vi "SeqWithMultichannel.vi"() -> ()   [LabVIEW 2014]
uses:
  <vilib>/Instr/_visa.llb/VISA Configure Serial Port (Instr).vi
panel:
  out "read buffer":string
  out "OutputStr":string
  in  "stop":bool
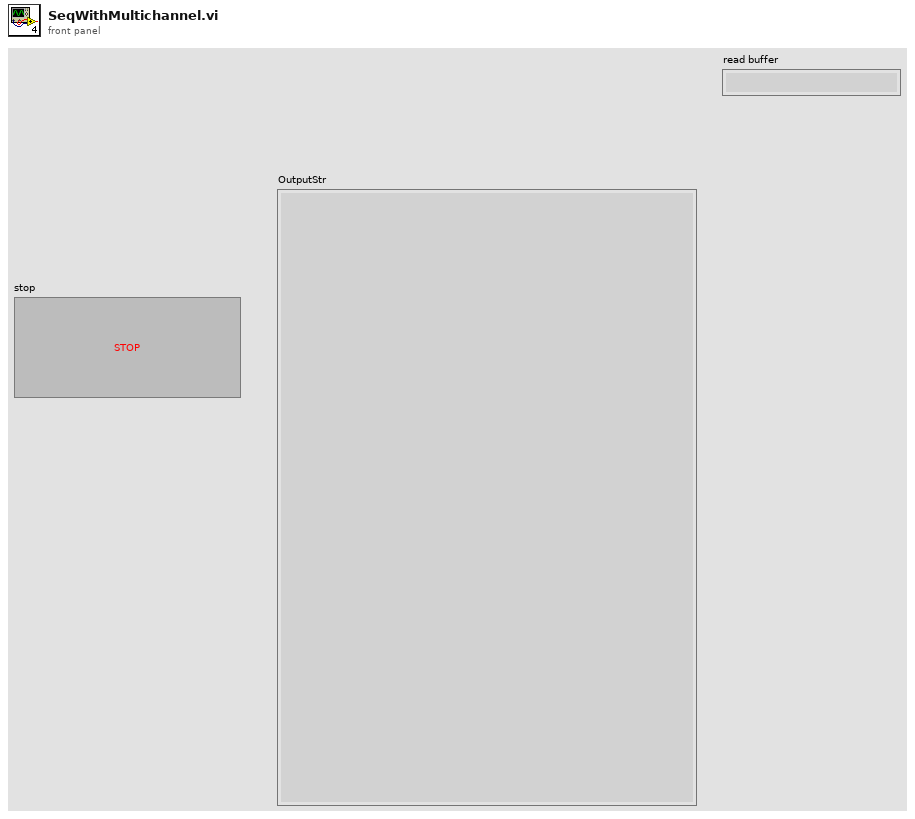
[diagram p1: front panel]
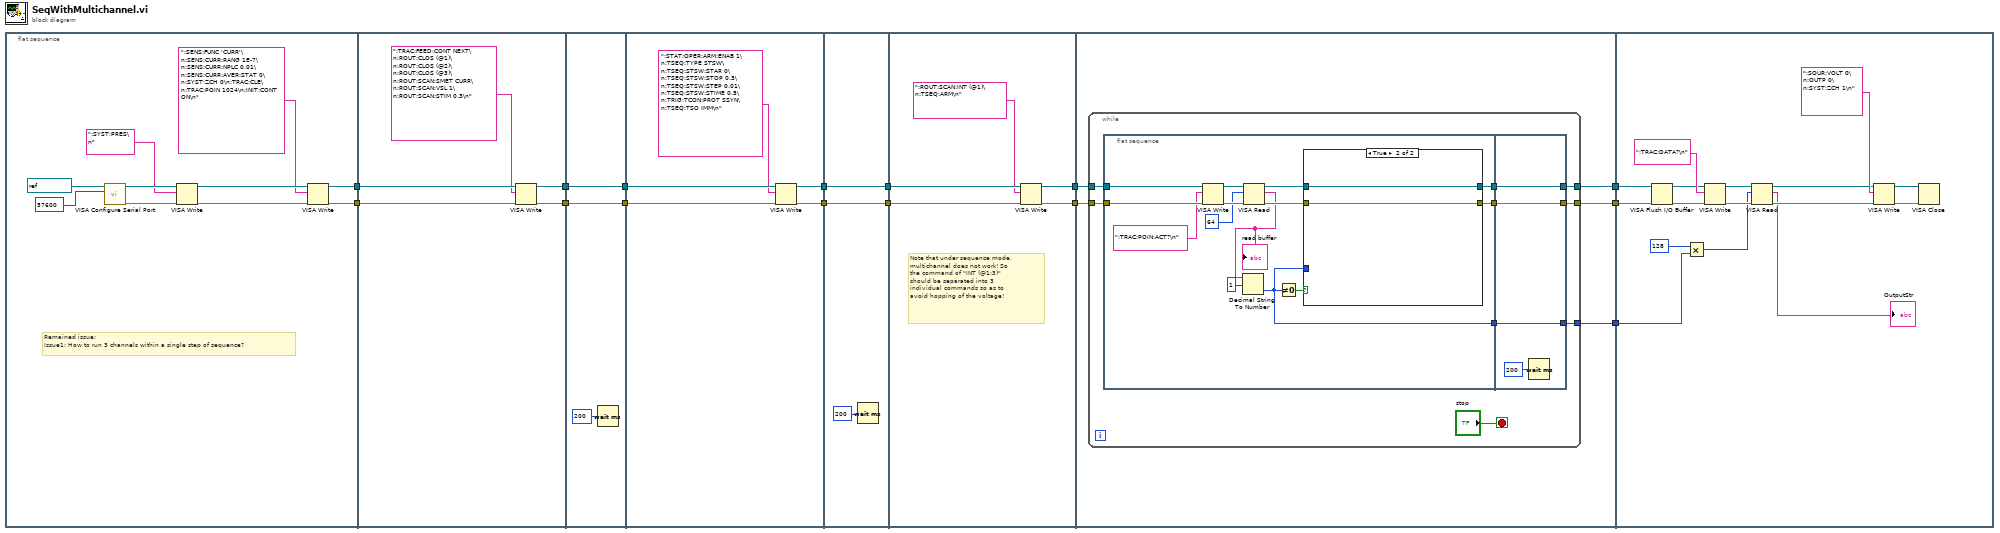
[diagram p0: block diagram]
diagram:
  n1 = flat-sequence {
    tunnel: [w17] -> w15
    tunnel: [w16] -> w14
    tunnel: w15 -> [w30]
    tunnel: w14 -> [w29]
    tunnel: [w27] -> w12
    tunnel: [w26] -> w10
    tunnel: [w32] -> w13
    tunnel: w12 -> [w32]
    tunnel: [w31] -> w11
    tunnel: w10 -> [w31]
    tunnel: w13 -> [w38]
    tunnel: w11 -> [w37]
    tunnel: [w35] -> w9
    tunnel: [w34] -> w7
    tunnel: w9 -> [w40]
    tunnel: [w41] -> w8
    tunnel: w7 -> [w41]
    tunnel: [w40] -> w6
    tunnel: w8 -> [w45]
    tunnel: w6 -> [w46]
    tunnel: [w43] -> w5
    tunnel: [w42] -> w4
    tunnel: w5 -> [w51]
    tunnel: w4 -> [w50]
    tunnel: [w49] -> w3
    tunnel: [w48] -> w2
    tunnel: [w47] -> w1
    tunnel: w3 -> [w86]
    tunnel: w2 -> [w85]
    tunnel: w1 -> [w90]
    frame #0 {
      # "Remained issue:\nIssue1: How to run 3 channels within a single step of sequence?"
      n2 = call-poly "VISA Configure Serial Port"("VISA resource name"=refnum<visa-resource-name> "COM8", "baud rate (9600)"=u32 57600) -> ("VISA resource name out"=w23:refnum<visa-resource-name>, "error out"=w22:errorcluster)  [unwired: 12 in]
      n3 = VISA Write(VISA resource name=w23, write buffer=":SYST:PRES\n", error in (no error)=w22) -> (VISA resource name out=w20:refnum<visa-resource-name>, error out=w19:errorcluster)  [unwired: 1 out]
      n4 = VISA Write(VISA resource name=w20, write buffer=":SENS:FUNC 'CURR'\n:SENS:CURR:RANG 1E-7\n:SENS:CURR:NPLC 0.01\n:SENS:CURR:AVER:STAT 0\n:SYST:ZCH 0\n:TRAC:CLE\n:TRAC:POIN 1024\n:INIT:CONT ON\n", error in (no error)=w19) -> (VISA resource name out=w17:refnum<visa-resource-name>, error out=w16:errorcluster)  [unwired: 1 out]
    }
    frame #1 {
      n5 = VISA Write(VISA resource name=w30, write buffer=":TRAC:FEED:CONT NEXT\n:ROUT:CLOS (@1)\n:ROUT:CLOS (@2)\n:ROUT:CLOS (@3)\n:ROUT:SCAN:SMET CURR\n:ROUT:SCAN:VSL 1\n:ROUT:SCAN:STIM 0.3\n", error in (no error)=w29) -> (VISA resource name out=w27:refnum<visa-resource-name>, error out=w26:errorcluster)  [unwired: 1 out]
    }
    frame #2 {
      n6 = Wait (ms)(milliseconds to wait=u32 200) -> ()  [unwired: 1 out]
    }
    frame #3 {
      n7 = VISA Write(VISA resource name=w38, write buffer=":STAT:OPER:ARM:ENAB 1\n:TSEQ:TYPE STSW\n:TSEQ:STSW:STAR 0\n:TSEQ:STSW:STOP 0.3\n:TSEQ:STSW:STEP 0.01\n:TSEQ:STSW:STIME 0.5\n:TRIG:TCON:PROT SSYN\n:TSEQ:TSO IMM\n", error in (no error)=w37) -> (VISA resource name out=w35:refnum<visa-resource-name>, error out=w34:errorcluster)  [unwired: 1 out]
    }
    frame #4 {
      n8 = Wait (ms)(milliseconds to wait=u32 200) -> ()  [unwired: 1 out]
    }
    frame #5 {
      # "Note that under sequence mode, \nmultichannel does not work! So \nthe command of \"INT (@1:3)\" \nshould be separated into 3 \nindividual commands so as to \navoid hopping of the voltage!"
      n9 = VISA Write(VISA resource name=w46, write buffer=":ROUT:SCAN:INT (@1)\n:TSEQ:ARM\n", error in (no error)=w45) -> (VISA resource name out=w43:refnum<visa-resource-name>, error out=w42:errorcluster)  [unwired: 1 out]
    }
    frame #6 {
      n10 = while {
        tunnel: w51 -> [w59]
        tunnel: w50 -> [w58]
        tunnel: [w55] -> w49
        tunnel: [w54] -> w48
        tunnel: [w52] -> w47
        stop <- "stop" stop-if-true
        n11 = flat-sequence {
          tunnel: w59 -> [w74]
          tunnel: w58 -> [w73]
          tunnel: [w63] -> w57
          tunnel: [w62] -> w56
          tunnel: [w61] -> w53
          tunnel: w57 -> [w81]
          tunnel: w56 -> [w80]
          tunnel: [w81] -> w55
          tunnel: [w80] -> w54
          tunnel: [w79] -> w52
          tunnel: w53 -> [w79]
          frame #0 {
            n12 = VISA Write(VISA resource name=w74, write buffer=":TRAC:POIN:ACT?\n", error in (no error)=w73) -> (VISA resource name out=w71:refnum<visa-resource-name>, error out=w70:errorcluster)  [unwired: 1 out]
            n13 = VISA Read(VISA resource name=w71, byte count=u32 64, error in (no error)=w70) -> (VISA resource name out=w68:refnum<visa-resource-name>, read buffer=w66:string, error out=w67:errorcluster)  [unwired: 1 out]
            "read buffer" <- w66
            n14 = Decimal String To Number(string=w66, offset=1) -> (number=w61:i32)  [unwired: 1 in, 1 out]
            n15 = Not Equal To 0?(x=w61) -> (x != 0?=w64:bool)
            n16 = case shown="True" w64 {
              tunnel: w68 -> [w76 w78]
              tunnel: w67 -> [w75 w77]
              tunnel: w61 -> [_ _]
              tunnel: [w76 w78] -> w63
              tunnel: [w75 w77] -> w62
              frame False {
              }
              frame True {
              }
            }
          }
          frame #1 {
            n17 = Wait (ms)(milliseconds to wait=u32 200) -> ()  [unwired: 1 out]
          }
        }
      }
    }
    frame #7 {
      n18 = VISA Flush I/O Buffer(VISA resource name=w86, error in (no error)=w85) -> (VISA resource name out=w84:refnum<visa-resource-name>, error out=w83:errorcluster)  [unwired: 1 in]
      n19 = Multiply(x=128, y=w90) -> (x*y=w92:i32)
      n20 = VISA Write(VISA resource name=w84, write buffer=":TRAC:DATA?\n", error in (no error)=w83) -> (VISA resource name out=w93:refnum<visa-resource-name>, error out=w94:errorcluster)  [unwired: 1 out]
      n21 = VISA Read(VISA resource name=w93, byte count=w92, error in (no error)=w94) -> (VISA resource name out=w89:refnum<visa-resource-name>, read buffer=→"OutputStr":string, error out=w88:errorcluster)  [unwired: 1 out]
      n22 = VISA Write(VISA resource name=w89, write buffer=":SOUR:VOLT 0\n:OUTP 0\n:SYST:ZCH 1\n", error in (no error)=w88) -> (VISA resource name out=w97:refnum<visa-resource-name>, error out=w96:errorcluster)  [unwired: 1 out]
      n23 = VISA Close(VISA resource name=w97, error in (no error)=w96) -> ()  [unwired: 1 out]
    }
  }
